vi "DHT22_readhumidity.vi"() -> ()   [LabVIEW 2014]
uses:
  <vilib>/Instr/_visa.llb/VISA Configure Serial Port (Instr).vi
panel:
  out "Humidity (%) 2":cluster{dbl}(graph)
  out "temp (C)":string
  out "humidity (%)":string
  out "gas sensor":string
  in  "Arduino":bool
  out "read buffer":string
  in  "stop":bool
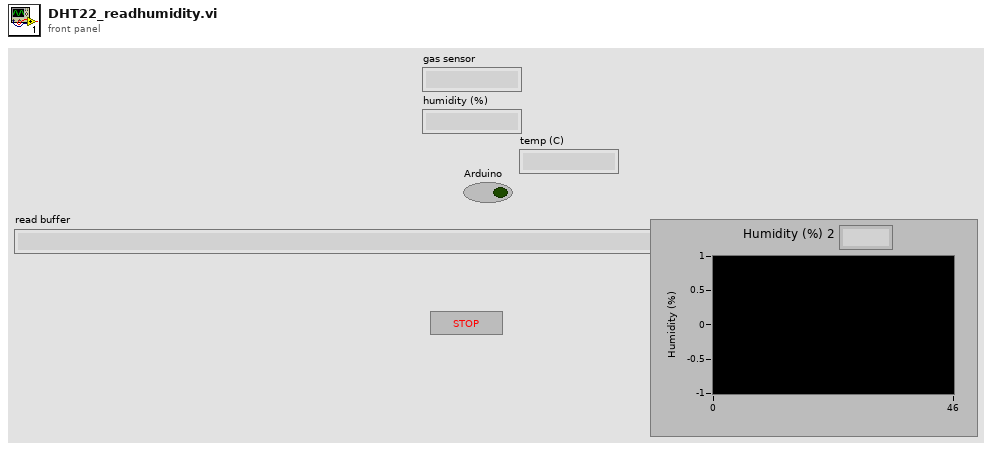
[diagram p1: front panel]
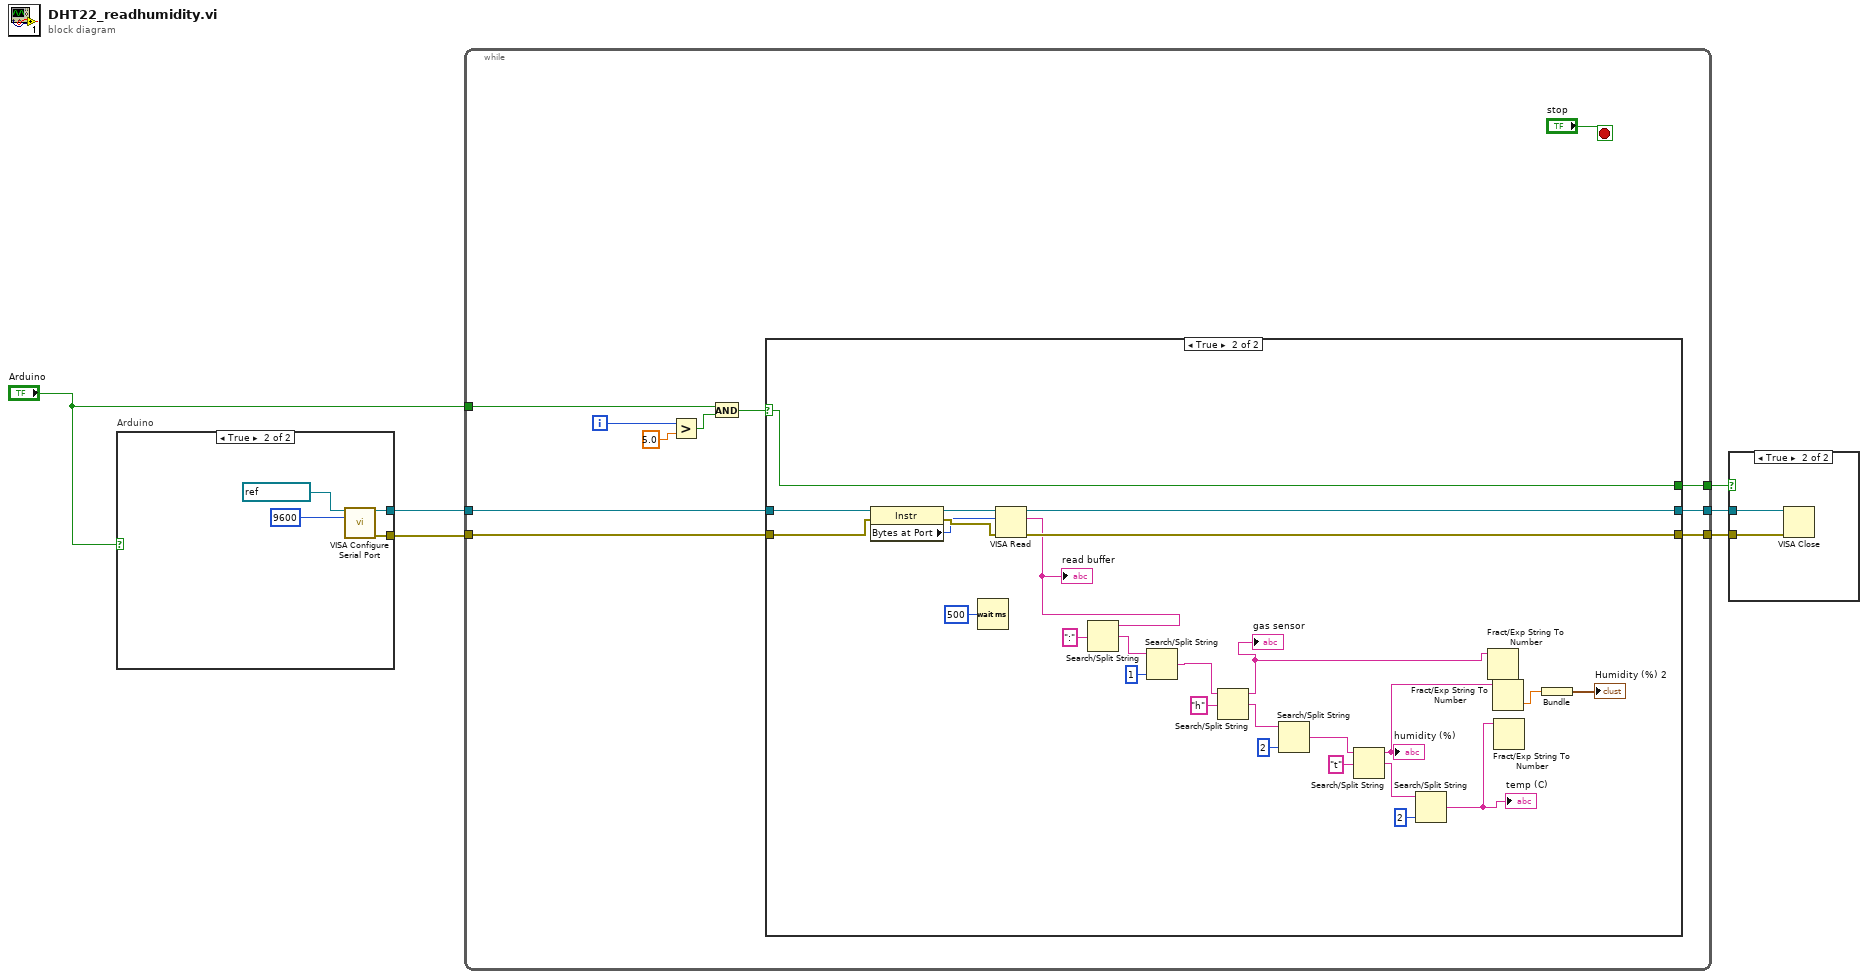
[diagram p0: block diagram]
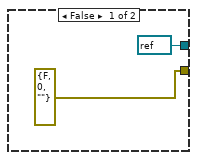
[diagram p3: hidden frame]
diagram:
  n1 = case "Arduino" shown="True" "Arduino" {
    tunnel: [refnum<visa-resource-name> refnum ("VISA resource name out") w12] -> w4
    tunnel: [errorcluster {"status"=FALSE, "code"=0, "source"=""} ("error out") w9] -> w3
    frame False {
    }
    frame True {
      n2 = call-poly "VISA Configure Serial Port"("VISA resource name"=refnum<visa-resource-name> "COM12", "baud rate (9600)"=u32 9600) -> ("VISA resource name out"=w12:refnum<visa-resource-name>, "error out"=w9:errorcluster)  [unwired: 12 in]
    }
  }
  n3 = while {
    tunnel: w4 -> [w15]
    tunnel: w3 -> [w14]
    tunnel: [w22] -> w6
    tunnel: [w21] -> w5
    tunnel: "Arduino" -> [w17]
    tunnel: [w13] -> w1
    i -> [w19]
    stop <- "stop" stop-if-true
    n4 = Greater?(x=w19, y=5.0) -> (0:w18:bool)
    n5 = And(x=w17, y=w18) -> (x .and. y?=w16:bool)
    n6 = case shown="True" w16 {
      selector: w16 -> [w24 w45]
      tunnel: w15 -> [w26 w49]
      tunnel: w14 -> [w25 w48]
      tunnel: [w26 w46] -> w22
      tunnel: [w25 w47] -> w21
      tunnel: [w24 w45] -> w13
      frame False {
      }
      frame True {
        n7 = property class="Instr"(reference=w49, error in=w48) -> (reference out=w50:refnum<visa-resource-name>, error out=w52:errorcluster, "Bytes at Port"=w51:u32)
        n8 = Wait (ms)(milliseconds to wait=u32 500) -> ()  [unwired: 1 out]
        n9 = VISA Read(VISA resource name=w50, byte count=w51, error in (no error)=w52) -> (VISA resource name out=w46:refnum<visa-resource-name>, read buffer=w42:string, error out=w47:errorcluster)  [unwired: 1 out]
        "read buffer" <- w42
        n10 = Search/Split String(string=w42, search string/char (-)=":") -> (match + rest of string=w40:string)  [unwired: 1 in, 2 out]
        n11 = Search/Split String(string=w40, offset (0)=1) -> (match + rest of string=w38:string)  [unwired: 1 in, 2 out]
        n12 = Search/Split String(string=w38, search string/char (-)="h") -> (substring before match=w31:string, match + rest of string=w36:string)  [unwired: 1 in, 1 out]
        "gas sensor" <- w31
        n13 = Search/Split String(string=w36, offset (0)=2) -> (match + rest of string=w34:string)  [unwired: 1 in, 2 out]
        n14 = Search/Split String(string=w34, search string/char (-)="t") -> (substring before match=w30:string, match + rest of string=w32:string)  [unwired: 1 in, 1 out]
        "humidity (%)" <- w30
        n15 = Search/Split String(string=w32, offset (0)=2) -> (match + rest of string=w29:string)  [unwired: 1 in, 2 out]
        "temp (C)" <- w29
        n16 = Fract/Exp String To Number(string=w31) -> ()  [unwired: 3 in, 2 out]
        n17 = Fract/Exp String To Number(string=w30) -> (number=w27:dbl)  [unwired: 3 in, 1 out]
        n18 = Fract/Exp String To Number(string=w29) -> ()  [unwired: 3 in, 2 out]
        n19 = Bundle(w27) -> (→"Humidity (%) 2":cluster{dbl})  [unwired: 1 in]
      }
    }
  }
  n20 = case shown="True" w1 {
    tunnel: w6 -> [_ w54]
    tunnel: w5 -> [_ w53]
    frame False {
    }
    frame True {
      n21 = VISA Close(VISA resource name=w54, error in (no error)=w53) -> ()  [unwired: 1 out]
    }
  }
